vi "画路径线条.vi"(7 "图片输入":picture, 8 "结束行":i32=1, 9 "结束列":i32=1, 10 "开始行":i32=1, 11 "开始列":i32=1) -> (3 "图片输出":picture)   [LabVIEW 2020]
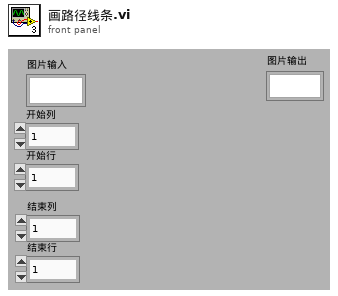
[diagram p1: front panel]
types:
  T1 = cluster{"Width":u16, "Style":enum32{"Solid", "Dash", "Dot", "DashDot", "DashDotDot"}}
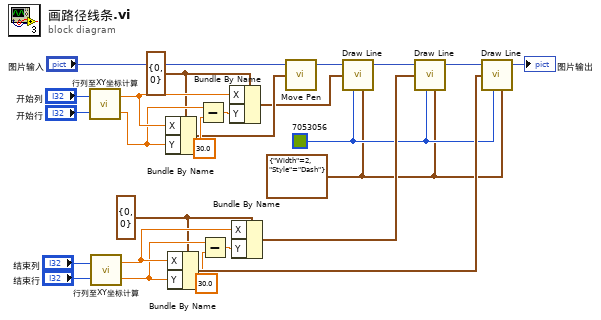
[diagram p0: block diagram]
diagram:
  w10 = cluster{"X":i32, "Y":i32} {"X"=0, "Y"=0} ("Mouse Position")
  w1 = T1 {"Width"=2, "Style"=enum."Dash"} ("pen")
  w2 = u32 7053056 ("color(black)")
  w15 = cluster{"X":i32, "Y":i32} {"X"=0, "Y"=0} ("Mouse Position")
  n1 = call "行列至XY坐标计算.vi"("行位置"="开始行", "列位置"="开始列") -> ("纵坐标"=w11:dbl, "横坐标"=w12:dbl)
  n2 = call "行列至XY坐标计算.vi"("行位置"="结束行", "列位置"="结束列") -> ("纵坐标"=w17:dbl, "横坐标"=w24:dbl)
  n3 = Bundle By Name(cluster=w10, "X"=w12, "Y"=w11) -> (w7:cluster{"X":i32, "Y":i32})
  n4 = Bundle By Name(cluster=w15, "X"=w24, "Y"=w17) -> (w25:cluster{"X":i32, "Y":i32})
  n5 = Subtract(x=w11, y=30.0) -> (x-y=w14:dbl)
  n6 = Subtract(x=w17, y=30.0) -> (x-y=w23:dbl)
  n7 = Bundle By Name(cluster=w10, "X"=w12, "Y"=w14) -> (w6:cluster{"X":i32, "Y":i32})
  n8 = Bundle By Name(cluster=w15, "X"=w24, "Y"=w23) -> (w3:cluster{"X":i32, "Y":i32})
  n9 = call <vilib>:"Move Pen.vi"("new position"=w7, "picture"="图片输入") -> ("new picture"=w8:picture)  [unwired: 3 in]
  n10 = call <vilib>:"Draw Line.vi"("picture"=w8, "end point"=w6, "color(black)"=w2, "pen"=w1) -> ("new picture"=w5:picture)  [unwired: 5 in]
  n11 = call <vilib>:"Draw Line.vi"("picture"=w5, "end point"=w3, "color(black)"=w2, "pen"=w1) -> ("new picture"=w4:picture)  [unwired: 5 in]
  n12 = call <vilib>:"Draw Line.vi"("picture"=w4, "end point"=w25, "color(black)"=w2, "pen"=w1) -> ("new picture"=→"图片输出":picture)  [unwired: 5 in]
